vi "Fire Detection LabView.vi"() -> ()   [LabVIEW 2020]
panel:
  in  "Table Control":string[][](table)
  in  "VISA resource name":refnum<visa-resource-name>
  out "TEMP":dbl(graph)
  out "FIRE":dbl(graph)
  out "SMOKE":dbl(graph)
  out "FIRE":bool
  out "FLAME Indicator":bool
  out "SMOKE Indicator":bool
  out "FIRE METER":dbl(knob) scale=0.0..10.0
  out "SMOKE METER":dbl(knob) scale=0.0..10.0
  out "Temperature":dbl(slide) scale=0.0..100.0
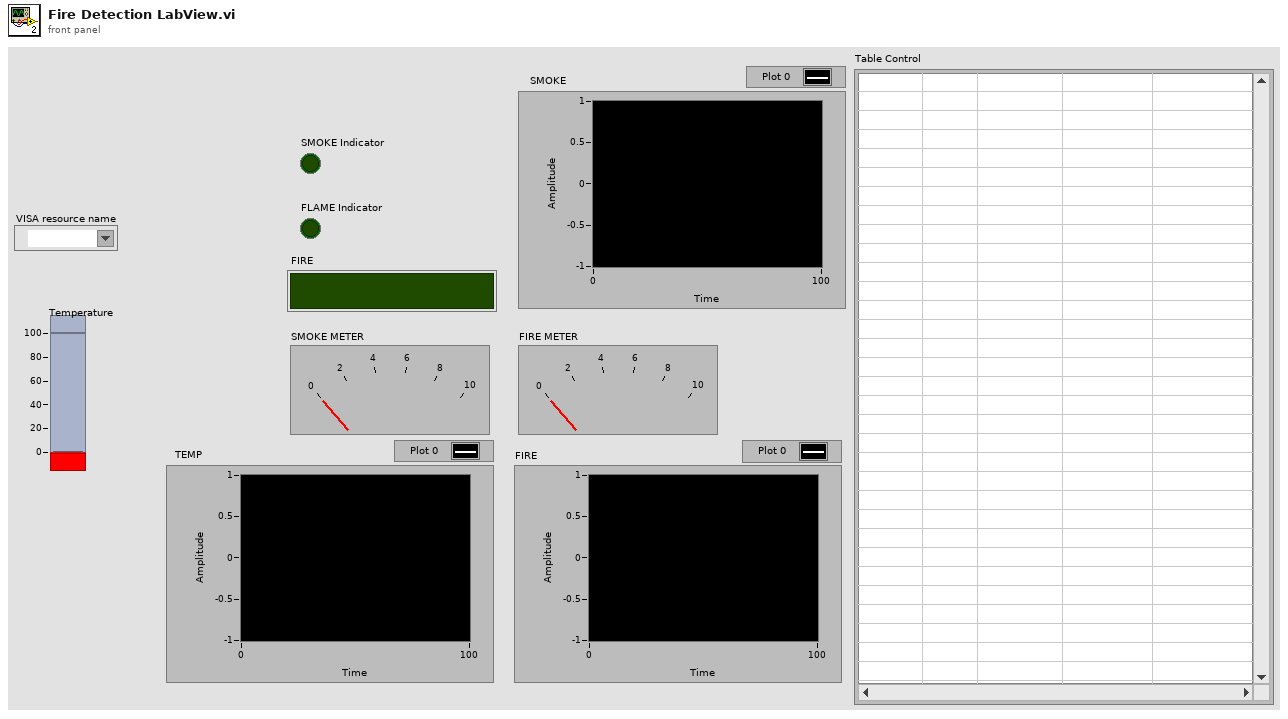
[diagram p1: front panel]
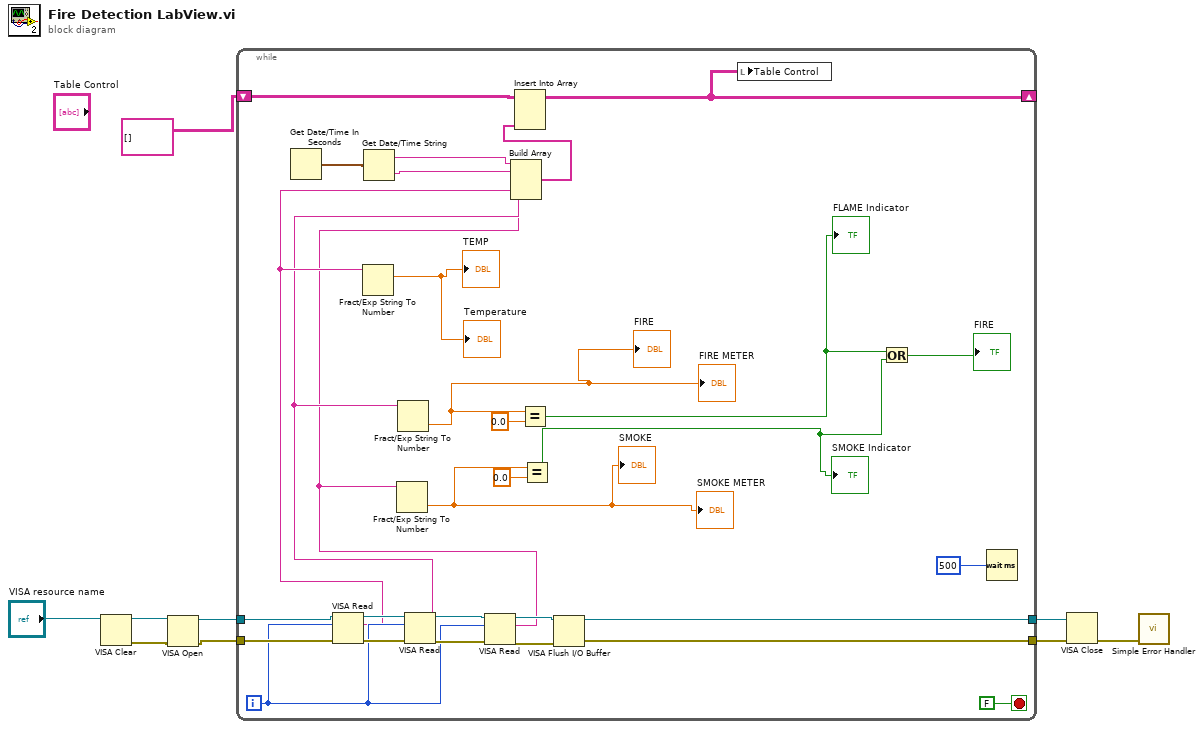
[diagram p0: block diagram]
diagram:
  n1 = VISA Clear(VISA resource name="VISA resource name") -> (VISA resource name out=w8:refnum<visa-resource-name>, error out=w7:errorcluster)  [unwired: 1 in]
  n2 = VISA Open(error in (no error)=w7, VISA resource name=w8) -> (VISA resource name=w6:refnum<visa-resource-name>, error out=w5:errorcluster)  [unwired: 3 in]
  n3 = while {
    shift-right: [w26] -> _
    shift-left: string[][] [] -> [w27]
    tunnel: w6 -> [w38]
    tunnel: w5 -> [w37]
    tunnel: [w30] -> w4
    tunnel: [w29] -> w3
    i -> [w28]
    stop <- FALSE stop-if-true
    n4 = Get Date/Time In Seconds() -> (seconds since 1Jan1904=w25:timestamp)
    n5 = VISA Read(VISA resource name=w38, byte count=w28, error in (no error)=w37) -> (VISA resource name out=w36:refnum<visa-resource-name>, read buffer=w22:string, error out=w35:errorcluster)  [unwired: 1 out]
    n6 = Fract/Exp String To Number(string=w22) -> (number=→"Temperature" →"TEMP":dbl)  [unwired: 3 in, 1 out]
    n7 = Get Date/Time String(seconds (now)=w25) -> (date string=w24:string, time string=w23:string)  [unwired: 2 in]
    n8 = VISA Read(VISA resource name=w36, byte count=w28, error in (no error)=w35) -> (VISA resource name out=w34:refnum<visa-resource-name>, read buffer=w21:string, error out=w33:errorcluster)  [unwired: 1 out]
    n9 = Fract/Exp String To Number(string=w21) -> (number=w13:dbl)  [unwired: 3 in, 1 out]
    "FIRE METER" <- w13
    "FIRE" <- w13
    n10 = VISA Read(VISA resource name=w34, byte count=w28, error in (no error)=w33) -> (VISA resource name out=w32:refnum<visa-resource-name>, read buffer=w20:string, error out=w31:errorcluster)  [unwired: 1 out]
    n11 = Fract/Exp String To Number(string=w20) -> (number=w12:dbl)  [unwired: 3 in, 1 out]
    "SMOKE METER" <- w12
    "SMOKE" <- w12
    n12 = Build Array(w24, w23, w22, w21, w20) -> (w11:string[])
    n13 = Insert Into Array(array=w27, new element=w11) -> (w26:string[][])  [unwired: 2 in]
    n14 = Equal?(x=w13, y=0.0) -> (x = y?=w16:bool)
    "FLAME Indicator" <- w16
    n15 = Equal?(x=w12, y=0.0) -> (x = y?=w15:bool)
    "SMOKE Indicator" <- w15
    n16 = VISA Flush I/O Buffer(VISA resource name=w32, error in (no error)=w31) -> (VISA resource name out=w30:refnum<visa-resource-name>, error out=w29:errorcluster)  [unwired: 1 in]
    n17 = local write "Table Control"(w26) -> ()
    n18 = Or(x=w16, y=w15) -> (x .or. y?=→"FIRE":bool)
    n19 = Wait (ms)(milliseconds to wait=u32 500) -> ()  [unwired: 1 out]
  }
  n20 = VISA Close(VISA resource name=w4, error in (no error)=w3) -> (error out=w2:errorcluster)
  n21 = call <vilib>:"Simple Error Handler.vi"("error in (no error)"=w2) -> ()  [unwired: 4 in, 5 out]
